vi "Update Chart.vi"(8 "error in (no error)":errorcluster, 10 "Chart in":T1={"ChartName"="", "AntiAliasing"=0, "background"={"Color"={"Color"=0, "alpha"=76}, "HatchStyle"=76, "GradientStyle"=0}} {"background"."GradientStyle" items=["None", "LeftRight", "TopBottom", "Center", "DiagonalLeft", "DiagonalRight", "HorizontalCenter", "VerticalCenter"]; "background"."HatchStyle" items=["None", "BackwardDiagonal", "Cross", "DarkDownwardDiagonal", "DarkHorizontal", "DarkUpwardDiagonal", "DarkVertical", "DashedDownwardDiagonal", "DashedHorizontal", "DashedUpwardDiagonal", "DashedVertical", "DiagonalBrick", "DiagonalCross", "Divot", "DottedDiamond", "DottedGrid", "ForwardDiagonal", "Horizontal", "HorizontalBrick", "LargeCheckerBoard", "LargeConfetti", "LargeGrid", "LightDownwardDiagonal", "LightHorizontal", "LightUpwardDiagonal", "LightVertical", "NarrowHorizontal", "NarrowVertical", "OutlinedDiamond", "Percent05", "Percent10", "Percent20", "Percent25", "Percent30", "Percent40", "Percent50", "Percent60", "Percent70", "Percent75", "Percent80", "Percent90", "Plaid", "Shingle", "SmallCheckerBoard", "SmallConfetti", "SmallGrid", "SolidDiamond", "Sphere", "Trellis", "Vertical", "Wave", "Weave", "WideDownwardDiagonal", "WideUpwardDiagonal", "ZigZag"]; "background"."Color"."alpha" scale=0.0..255.0; "AntiAliasing" items=["None", "Text", "Graphics", "All"]}, 11 ".NET Refnum in":refnum<k24>) -> (0 "error out":errorcluster, 3 ".NET Refnum out":refnum<k24>)   [LabVIEW 2014, in "XMSChart.xctl"]
uses:
  XMSChart.xctl
  System.Windows.Forms.DataVisualization
  Controls/Chart.ctl
  Controls/Background.ctl
  Controls/Color.ctl
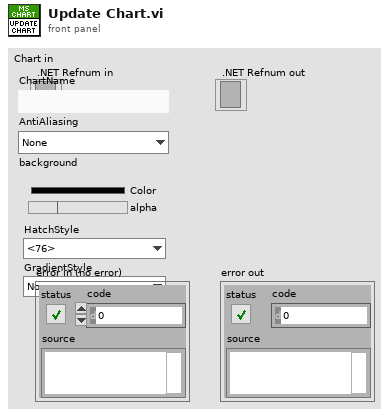
[diagram p1: front panel]
types:
  T1 = typedef "XMSChart.xctl/Chart.ctl" = cluster{"ChartName":string, "AntiAliasing":i32, "background":T2}
  T2 = typedef "XMSChart.xctl/Background.ctl" = cluster{"Color":T3, "HatchStyle":i32, "GradientStyle":i32}
  T3 = typedef "XMSChart.xctl/Color.ctl" = cluster{"Color":u32, "alpha":u8}
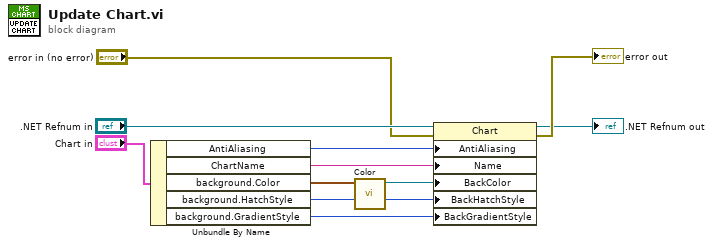
[diagram p0: block diagram]
diagram:
  n1 = Unbundle By Name("Chart in") -> ("AntiAliasing"=w5:i32, "ChartName"=w9:string, "background.Color"=w3:T3, "background.HatchStyle"=w2:i32, "background.GradientStyle"=w1:i32)
  n2 = call "Color.vi"("BGK Color"=w3) -> (".NET Refnum out"=w4:refnum<k24>)  [unwired: 10 in]
  n3 = property on="Property Node" class="Chart"(reference=".NET Refnum in", error in="error in (no error)", "AntiAliasing"=w5, "Name"=w9, "BackColor"=w4, "BackHatchStyle"=w2, "BackGradientStyle"=w1) -> (reference out=→".NET Refnum out":refnum<k24>, error out=→"error out":errorcluster)
